vi "Parse Config File.vi"(8 "error in (no error)":errorcluster, 9 "Protocol Type in":T1, 10 "Config File":path, 11 "File Parser Interface in":refnum<class "File Parser Interface.lvclass">) -> (0 "error out":errorcluster, 1 "Protocol Type out":T1, 2 "Config Array":string[](array[string]), 3 "File Parser Interface out":refnum<class "File Parser Interface.lvclass">)   [LabVIEW 2018, in "File Parser Interface.lvlib" / "File Parser Interface.lvclass"]
uses:
  File Parser Interface.lvclass
  Ctls/Protocol Type.ctl
  File Parser Interface.lvclass/File Parser Interface.ctl
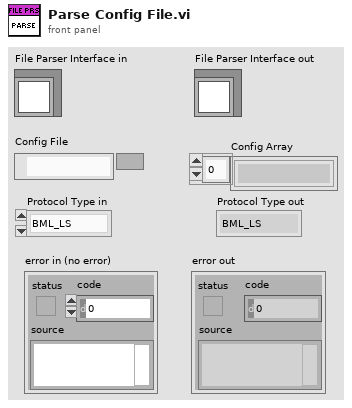
[diagram p1: front panel]
types:
  T1 = typedef "Protocol Type.ctl" = enum16{"BML_LS", "BML_HS", "SPI_3W", "SPI_4W"}
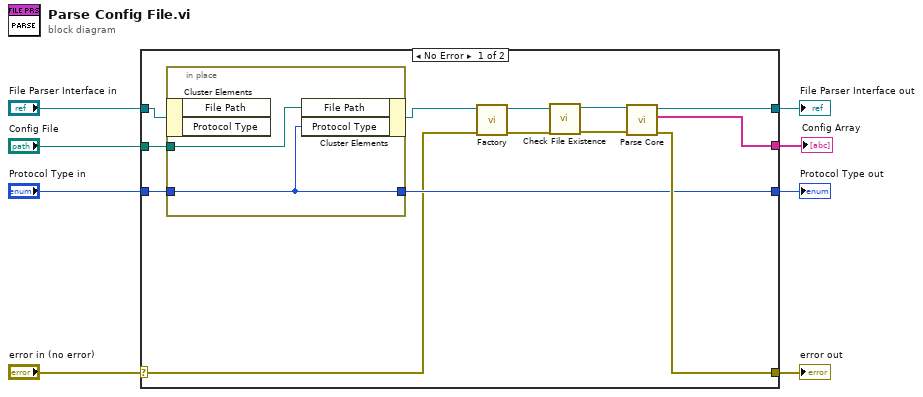
[diagram p0: block diagram]
diagram:
  n1 = case shown="No Error" "error in (no error)" {
    selector: "error in (no error)" -> [w12 w26]
    tunnel: [w17 w26] -> w7
    tunnel: [w19 w25] -> w5
    tunnel: "File Parser Interface in" -> [w21 w25]
    tunnel: "Config File" -> [w20 _]
    tunnel: [w18 _] -> w3
    tunnel: "Protocol Type in" -> [w14 w24]
    tunnel: [w13 w24] -> w1
    frame No Error {
      n2 = in-place {
        in-place-border: w20 -> [w23]
        in-place-border: w14 -> [w22]
        in-place-border: [w22] -> w13
        n3 = in-place-cluster #1(w21) -> ()  [unwired: 2 out]
        n4 = in-place-cluster #1("File Path"=w23, "Protocol Type"=w22) -> (w10:refnum<class "File Parser Interface.lvclass">)
      }
      n5 = call "Factory.vi"("error in (no error)"=w12, "File Parser Interface in"=w10) -> ("error out"=w11:errorcluster, "File Parser Interface out"=w9:refnum<class "File Parser Interface.lvclass">)  [unwired: 8 in]
      n6 = call "Check File Existence.vi"("error in (no error)"=w11, "File Parser Interface in"=w9) -> ("error out"=w16:errorcluster, "File Parser Interface out"=w15:refnum<class "File Parser Interface.lvclass">)  [unwired: 8 in]
      n7 = call-dynamic "Parse Core.vi"("error in (no error)"=w16, "File Parser Interface in"=w15) -> ("error out"=w17:errorcluster, "Config Array"=w18:string[], "File Parser Interface out"=w19:refnum<class "File Parser Interface.lvclass">)  [unwired: 7 in]
    }
    frame Error {
    }
  }
  "error out" <- w7
  "File Parser Interface out" <- w5
  "Config Array" <- w3
  "Protocol Type out" <- w1
